vi "Count Open Tabs.vi"(8 "error in":errorcluster, 11 "Tab Pages References In":refnum<vi>[](array[refnum])) -> (0 "error out":errorcluster, 2 "Number of Open Tabs":i32, 3 "Tab Pages References Out":refnum<vi>[](array[refnum]))   [LabVIEW 2017, in "DTacq Plot Display Library.lvlib"]
uses:
  DTacq Plot Display Library.lvlib
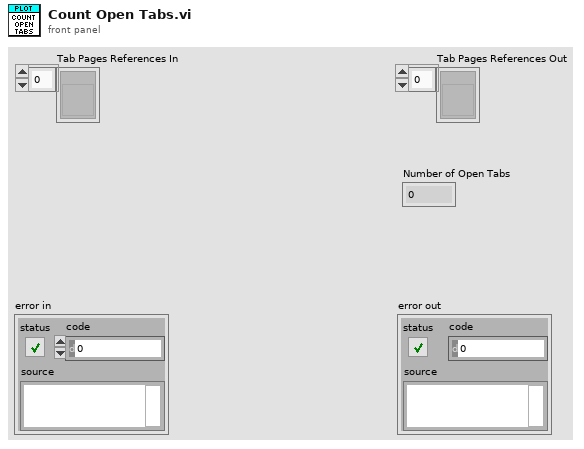
[diagram p1: front panel]
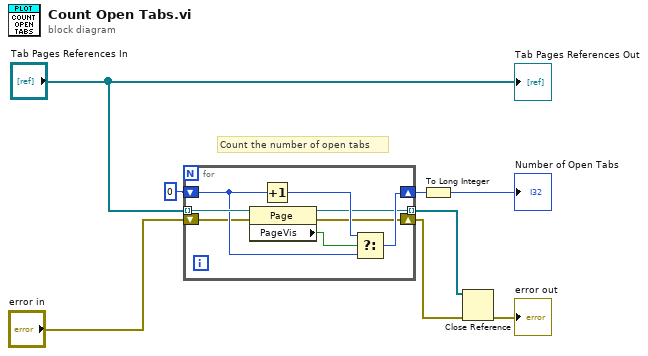
[diagram p0: block diagram]
diagram:
  # "Count the number of open tabs"
  n1 = for {
    tunnel: "Tab Pages References In" -> [w16] mode=indexing
    shift-right: [w12] -> w7
    shift-left: 0 -> [w13]
    tunnel: [w11] -> w4 mode=indexing
    shift-right: [w9] -> w2
    shift-left: "error in" -> [w10]
    n2 = property class="Page"(reference=w16, error in=w10) -> (reference out=w11:refnum<vi>, error out=w9:errorcluster, "PageVis"=w15:bool)
    n3 = Increment(x=w13) -> (x+1=w14:i32)
    n4 = Select(t=w14, s=w15, f=w13) -> (s? t:f=w12:i32)
  }
  n5 = To Long Integer(number=w7) -> (32bit integer=→"Number of Open Tabs":i32)
  n6 = Close Reference(reference=w4, error in (no error)=w2) -> (error out=→"error out":errorcluster)
  "Tab Pages References Out" <- "Tab Pages References In"
